vi "EnteringTextForGraph (SubVI).vi"(11 "Char":i16) -> (3 "Discard?":bool)   [LabVIEW 2017]
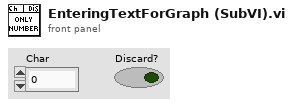
[diagram p1: front panel]
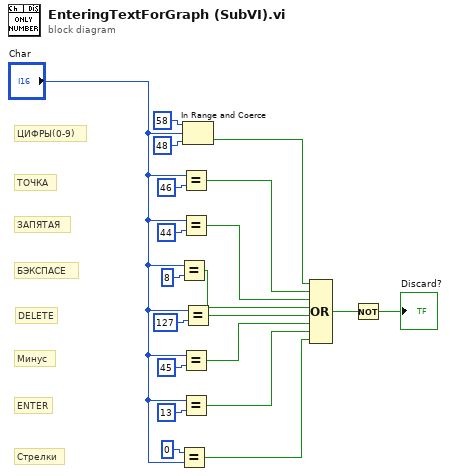
[diagram p0: block diagram]
diagram:
  # "Стрелки"
  # "ENTER"
  # "Минус"
  # "DELETE"
  # "БЭКСПАСЕ"
  # "ЗАПЯТАЯ"
  # "ТОЧКА"
  # "ЦИФРЫ(0-9)"
  n1 = Equal?(x="Char", y=i16 8 ("lower limit")) -> (x = y?=w14:bool)
  n2 = Equal?(x=i16 0 ("lower limit"), y="Char") -> (x = y?=w20:bool)
  n3 = Equal?(x="Char", y=i16 46 ("lower limit")) -> (x = y?=w12:bool)
  n4 = Equal?(x="Char", y=i16 44 ("lower limit")) -> (x = y?=w13:bool)
  n5 = Equal?(x="Char", y=i16 45 ("lower limit")) -> (x = y?=w16:bool)
  n6 = Equal?(x="Char", y=i16 13 ("lower limit")) -> (x = y?=w17:bool)
  n7 = In Range and Coerce(upper limit=i16 58, x="Char", lower limit=i16 48) -> (In Range?=w11:bool)  [unwired: 1 out]
  n8 = Equal?(x="Char", y=i16 127 ("lower limit")) -> (x = y?=w15:bool)
  n9 = Compound Arithmetic op=OR(w11, w12, w13, w14, w15, w16, w17, w20) -> (w9:bool)
  n10 = Not(x=w9) -> (.not. x?=→"Discard?":bool)
